vi "Create.vi"(7 "Skip Unload? (F)":bool, 8 "error in (no error)":errorcluster, 11 "SequenceFile":refnum<k7>) -> (0 "error out":errorcluster, 3 "SequenceFile out":refnum<class "SequenceFile.lvclass">)   [LabVIEW 2020, in "TSnax.lvlib" / "SequenceFile.lvclass"]
uses:
  SequenceFile.lvclass
  Ref Data.ctl
  PropertyObjectFile/PropertyObjectFile.lvclass
  PropertyObject/PropertyObject.lvclass
  SequenceFile.lvclass/SequenceFile.ctl
  TSnax.lvlib
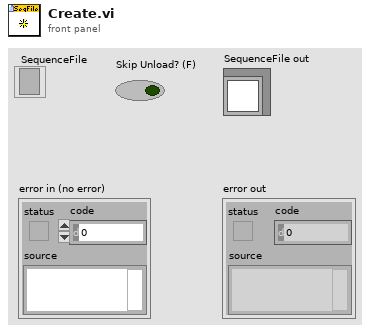
[diagram p1: front panel]
types:
  T1 = typedef "TSnax.lvlib/SequenceFile.lvclass/Ref Data.ctl" = cluster{"Process Model":refnum<class "PropertyObjectFile.lvclass">, "File Globals":refnum<class "PropertyObject.lvclass">}
  T2 = typedef "TSnax.lvlib/SequenceFile.lvclass/SequenceFile Type.ctl" = enum16{"Normal", "Model", "Front End Callbacks", "Station Callbacks", "Template"}
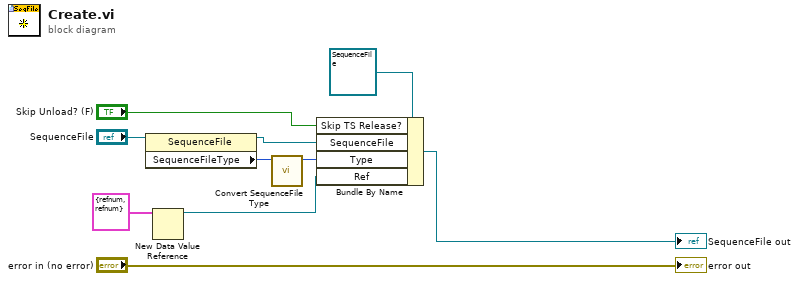
[diagram p0: block diagram]
diagram:
  n1 = property class="SequenceFile"(reference="SequenceFile") -> (reference out=w3:refnum<k7>, "SequenceFileType"=w6:i32)  [unwired: 1 in, 1 out]
  n2 = New Data Value Reference(data value=T1 {"Process Model"=refnum, "File Globals"=refnum} ("Ref Data")) -> (data value reference=w2:refnum<data-value>)  [unwired: 1 in, 1 out]
  n3 = call "Convert SequenceFile Type.vi"("TS API"=w6) -> ("TS API -> TSnax"=w5:T2)  [unwired: 9 in, 1 out]
  n4 = Bundle By Name(cluster=refnum<class "SequenceFile.lvclass"> refnum ("SequenceFile out"), "Skip TS Release?"="Skip Unload? (F)", "SequenceFile"=w3, "Type"=w5, "Ref"=w2) -> (→"SequenceFile out":refnum<class "SequenceFile.lvclass">)
  "error out" <- "error in (no error)"
